vi "Auto Elevator Finger.vi"(11 "Tote Count":i32) -> (3 "Boolean":bool)   [LabVIEW 2014]
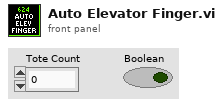
[diagram p1: front panel]
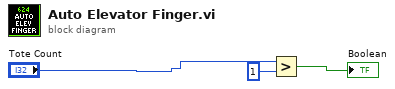
[diagram p0: block diagram]
diagram:
  n1 = Greater?(x="Tote Count", y=1) -> (0:→"Boolean":bool)
